vi "Oscilloscope Example.vi"() -> ()   [LabVIEW 2013]
uses:
  Panels_XControl/Panels_XControl.xctl
  UI Panels.lvlib
panel:
  in  "Stop":bool
  in  "UI Panels":refnum<vi>[](xcontrol)
  # "UI Panels, which can be\ncollapsed and expanded\nwith Dock/Undock functionality"
  # "Run this example (Ctrl+R)"
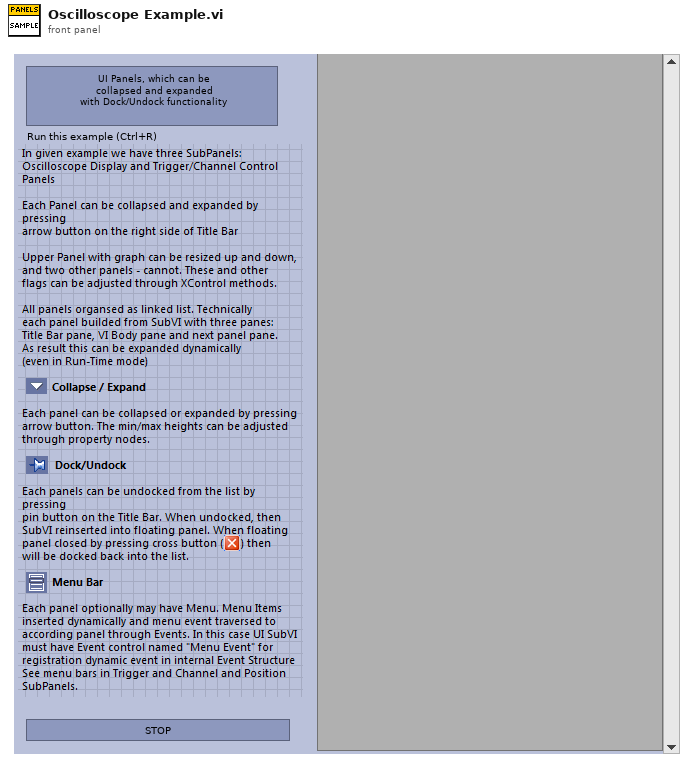
[diagram p1: front panel]
types:
  T1 = cluster{"Height (Collapsed)":i32, "Height (Collapsed) 2":i32}[]
  T2 = enum32{"invalid app kind", "Development System", "Run Time System", "Student Edition", "Embedded LabVIEW", "Evaluation", "Custom"}
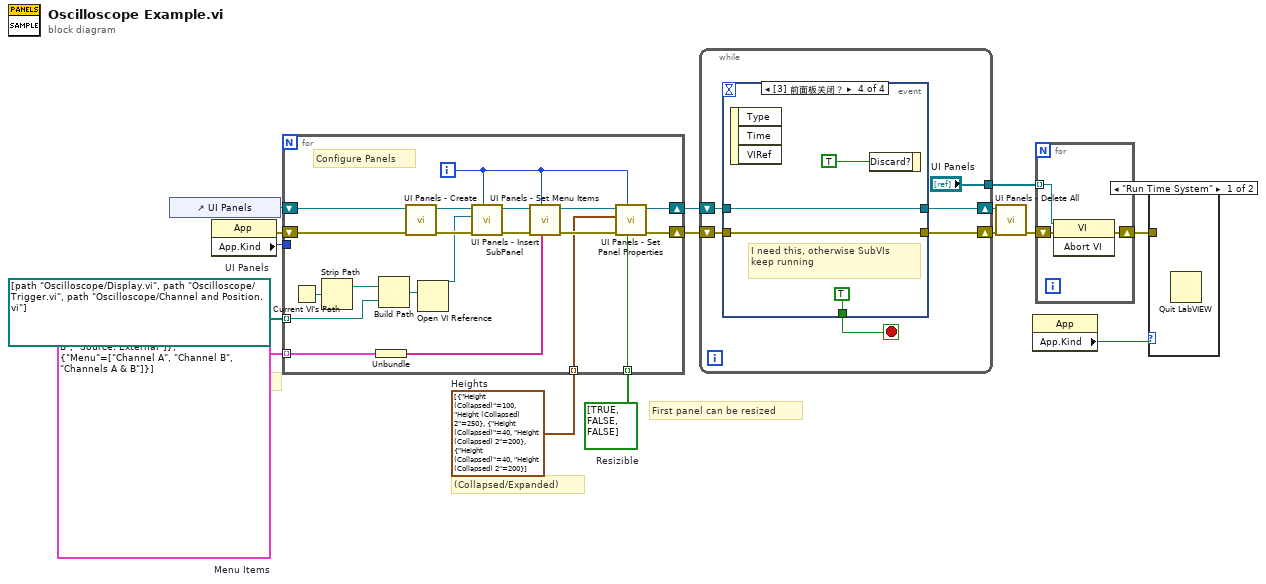
[diagram p0: block diagram]
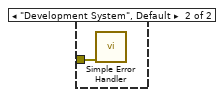
[diagram p2: hidden frame]
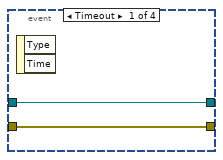
[diagram p3: hidden frame]
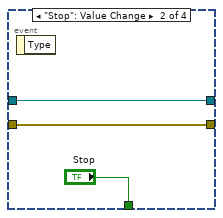
[diagram p4: hidden frame]
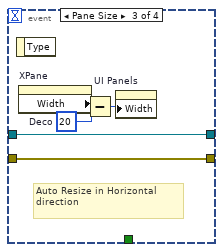
[diagram p5: hidden frame]
diagram:
  w2 = bool[] [TRUE, FALSE, FALSE]  # Resizible
  w3 = T1 [{"Height (Collapsed)"=100, "Height (Collapsed) 2"=250}, {"Height (Collapsed)"=40, "Height (Collapsed) 2"=200}, {"Height (Collapsed)"=40, "Height (Collapsed) 2"=200}]  # Heights
  w5 = cluster{"Menu":string[]}[] [{"Menu"=[]}, {"Menu"=["Source: Channel B", "Source: External"]}, {"Menu"=["Channel A", "Channel B", "Channels A & B"]}]  # Menu Items
  w15 = path[] [path "Oscilloscope/Display.vi", path "Oscilloscope/Trigger.vi", path "Oscilloscope/Channel and Position.vi"]  # UI Panels
  # "First Panel without menu"
  # "(Collapsed/Expanded)"
  # "First panel can be resized"
  n1 = control-ref of="UI Panels"() -> (w9:refnum<vi>)
  n2 = property class="App"() -> (error out=w7:errorcluster, "App.Kind"=w10:T2)  [unwired: 2 in, 1 out]
  n3 = for {
    tunnel: w15 -> [w24] mode=indexing
    shift-right: [w18] -> w6
    shift-left: w7 -> [w30]
    shift-right: [w21] -> w4
    shift-left: w9 -> [w33]
    tunnel: w10 -> [_]
    tunnel: w5 -> [w27] mode=indexing
    tunnel: w3 -> [w17] mode=indexing
    tunnel: w2 -> [w16] mode=indexing
    i -> [w25]
    # "Configure Panels"
    n4 = Current VI's Path() -> (path=w35:path)
    n5 = Strip Path(path=w35) -> (stripped path=w34:path)  [unwired: 1 out]
    n6 = Unbundle(w27) -> ("Menu"=w26:string[])
    n7 = Build Path(base path=w34, name or relative path=w24) -> (appended path=w28:path)
    n8 = call "UI Panels - Create.vi"("error in (no error)"=w30, "Panels_XControl"=w33) -> ("error out"=w31:errorcluster, "Panels_XControl"=w32:refnum<vi>)  [unwired: 8 in]
    n9 = Open VI Reference(vi path=w28) -> (vi reference=w29:refnum<vi>)  [unwired: 5 in, 1 out]
    n10 = call "UI Panels - Insert SubPanel.vi"("Panel index"=w25, "error in (no error)"=w31, "vi reference"=w29, "Panels_XControl"=w32) -> ("error out"=w20:errorcluster, "Panels_XControl"=w23:refnum<vi>)  [unwired: 6 in]
    n11 = call "UI Panels - Set Menu Items.vi"("Menu"=w26, "index"=w25, "error in (no error)"=w20, "Panels_XControl In"=w23) -> ("error out"=w19:errorcluster, "Panels_XControl Out"=w22:refnum<vi>)  [unwired: 6 in]
    n12 = call "UI Panels - Set Panel Properties.vi"("Resizible (T)"=w16, "index"=w25, "error in (no error)"=w19, "Height"=w17, "Panels_XControl"=w22) -> ("error out"=w18:errorcluster, "Panels_XControl Out"=w21:refnum<vi>)  [unwired: 5 in]
  }
  n13 = while {
    shift-right: [w40] -> w13
    shift-left: w4 -> [w39]
    shift-right: [w38] -> w12
    shift-left: w6 -> [w37]
    tunnel: ["UI Panels"] -> w14
    stop <- w41 stop-if-true
    n14 = event shown="[3] 前面板关闭？" {
      selector: _ -> [_ _ _ _]
      dyn-events: _ -> [_ _ _ _]
      timeout: _ -> [_ _ _ _]
      tunnel: [_ "Stop" _ TRUE ("Stop")] -> w41
      tunnel: [w43 w45 w51 w55] -> w40
      tunnel: w39 -> [w43 w45 w51 w55]
      tunnel: [w42 w44 w50 w54] -> w38
      tunnel: w37 -> [w42 w44 w50 w54]
      event Timeout {
        n15 = event-data() -> ()  [unwired: 1 in, 2 out]
      }
      event "Stop": Value Change {
        n16 = event-data() -> ()  [unwired: 1 in, 1 out]
      }
      event Pane Size {
        w47 = u32 20  # Deco
        # "Auto Resize in Horizontal\ndirection"
        n17 = event-data() -> ()  [unwired: 1 in, 1 out]
        n18 = property on="XPane" class="Pane"() -> ("Width"=w49:u32)  [unwired: 2 in, 2 out]
        n19 = Subtract(x=w49, y=w47) -> (x-y=w48:u32)
        n20 = property on="UI Panels" class="Panels_XControl (严格)"("Width"=w48) -> ()  [unwired: 2 in, 2 out]
      }
      event Panel Close? {
        # "I need this, otherwise SubVIs\nkeep running"
        n21 = event-data() -> ()  [unwired: 1 in, 3 out]
        n22 = event-data("Discard?"=TRUE) -> ()  [unwired: 1 in, 1 out]
      }
    }
  }
  n23 = call "UI Panels - Delete All.vi"("error in (No Error)"=w12, "Panels_XControl"=w13) -> ("error out"=w11:errorcluster)  [unwired: 8 in, 1 out]
  n24 = property class="App"() -> ("App.Kind"=w1:T2)  [unwired: 2 in, 2 out]
  n25 = for {
    tunnel: w14 -> [w58] mode=indexing
    shift-right: [w56] -> w8
    shift-left: w11 -> [w57]
    n26 = invoke class="VI" method="Abort VI"(reference=w58, error in=w57) -> (error out=w56:errorcluster)  [unwired: 1 in, 2 out]
  }
  n27 = case shown="\"Run Time System\"" w1 {
    tunnel: w8 -> [_ w59]
    frame "Run Time System" {
      n28 = Quit LabVIEW() -> ()  [unwired: 1 in]
    }
    frame "Development System", Default {
      n29 = call <vilib>:"Simple Error Handler.vi"("error in (no error)"=w59) -> ()  [unwired: 4 in, 5 out]
    }
  }
